vi "reset.vi"() -> ()   [LabVIEW 2022 SP3]
panel:
  out "InputReport1":u8[](array[numeric]) format="%x"
  out "Output Report":u8[](array[numeric])
  out "Input Report":u8[](array[numeric])
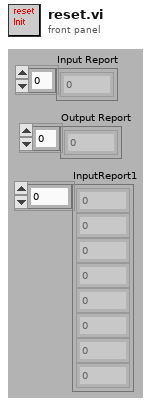
[diagram p1: front panel]
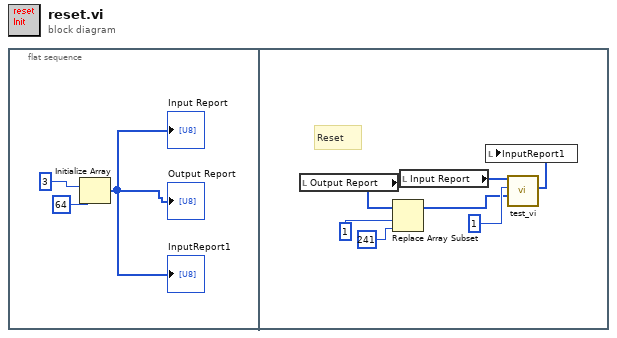
[diagram p0: block diagram]
diagram:
  n1 = flat-sequence {
    frame #0 {
      n2 = Initialize Array(u8 3 ("element"), 64 ("dimension size")) -> (→"Input Report" →"Output Report" →"InputReport1":u8[])
    }
    frame #1 {
      # "Reset"
      n3 = local read "Output Report"() -> (w6:u8[])
      n4 = Replace Array Subset(array=w6, new element=u8 241 ("new element/subarray"), index=1) -> (w5:u8[])
      n5 = local read "Input Report"() -> (w7:u8[])
      n6 = call "test_vi.vi"("OutputReport_in"=w5, "DevDet_in"=1, "InputReport_in"=w7) -> ("InputReport_out"=w4:u8[])  [unwired: 1 in, 3 out]
      n7 = local write "InputReport1"(w4) -> ()
    }
  }
